vi "Enable Close Outlet.vi"(0 "FPGA API in":refnum<class "FPGA API Concrete.lvclass">, 11 "error in (no error)":errorcluster, 13 "Direction":T1=enum."Chamber") -> (4 "FPGA API out":refnum<class "FPGA API Concrete.lvclass">, 15 "error out":errorcluster)   [LabVIEW 2019, in "FPGA API Concrete.lvclass"]
uses:
  FPGA API Concrete.lvclass
  TypeDef/Direction.ctl
  FPGA API Concrete.lvclass/FPGA API Concrete.ctl
  <vilib>/Utility/error.llb/Error Cluster From Error Code.vi
  <vilib>/rvi/errors/niLvFpgaAdjustHostInterfaceError.vi
  <vilib>/rvi/interface/nirviReadWriteControl/nirviReadWriteControl.xnode
  FPGA Ref.ctl
  NiFpgaLv.dll
  <vilib>/rvi/interface/Simulation/niFpgaSimulationCallBeginRW.vi
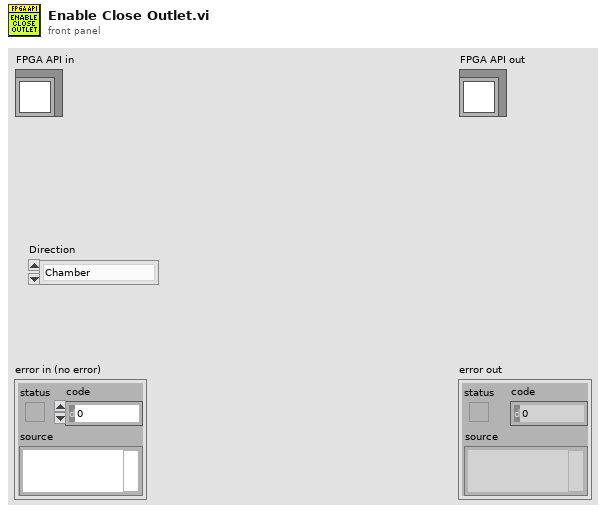
[diagram p1: front panel]
types:
  T1 = typedef "Direction.ctl" = enum16{"None", "Chamber", "DUT"}
  T2 = typedef "FPGA API Concrete.lvclass/FPGA Ref.ctl" = refnum<k20>
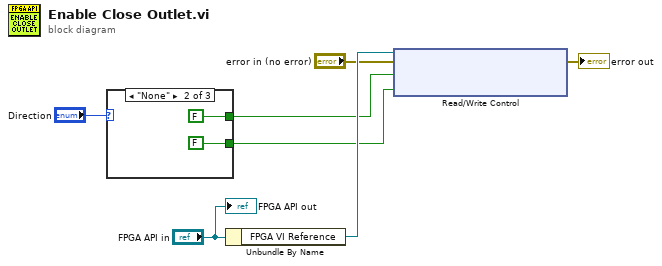
[diagram p0: block diagram]
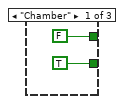
[diagram p2: hidden frame]
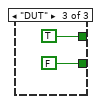
[diagram p3: hidden frame]
diagram:
  n1 = case shown="\"None\"" "Direction" {
    tunnel: [FALSE ("Enable Close Inlet") FALSE ("Enable Close Inlet") TRUE ("Enable Close Inlet")] -> w2
    tunnel: [TRUE ("Enable Close Inlet") FALSE ("Enable Close Inlet") FALSE ("Enable Close Inlet")] -> w1
    frame "Chamber" {
    }
    frame "None" {
    }
    frame "DUT" {
    }
  }
  n2 = Unbundle By Name("FPGA API in") -> ("FPGA VI Reference"=w6:T2)
  n3 = xnode "Read/Write Control"("FPGA VI Reference In"=w6, "error in"="error in (no error)", "Enable Close Outlet DUT"=w2, "Enable Close Outlet Chamber"=w1) -> ("error out"=→"error out":errorcluster)  [unwired: 1 out]
  "FPGA API out" <- "FPGA API in"
